vi "Recieve Idot Result utility.vi"(6 "Shots file":path=path "Z:/ShotHistory2014.txt", 7 "Log file folder":path=path "C:/Data/Shot Log.txt", 8 "error in (no error)":errorcluster, 10 "file path":path, 11 "Root Data Folder":path=path "C:/Data") -> (0 "error out":errorcluster, 2 "Formated shot data":string, 3 "File Path output":path)   [LabVIEW 2015]
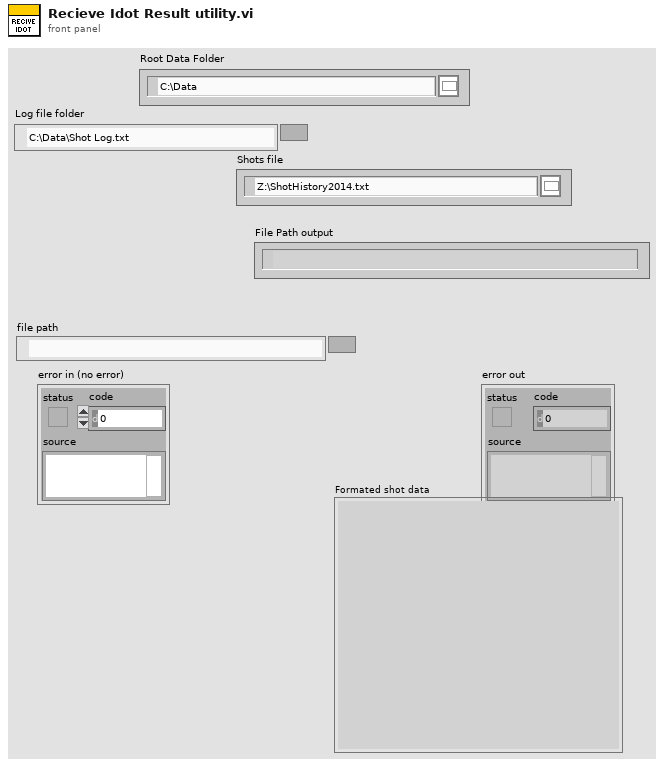
[diagram p1: front panel]
types:
  T1 = cluster{"file path":path, "Current time":timestamp, i32, dbl}
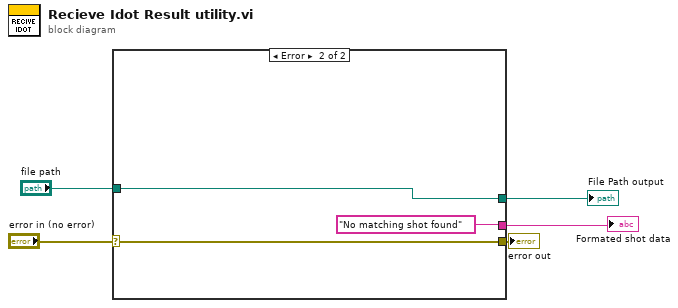
[diagram p0: block diagram]
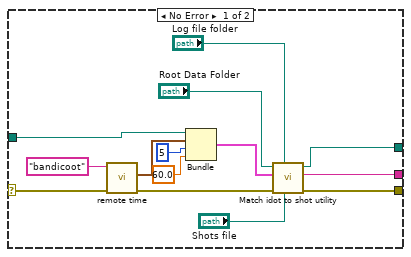
[diagram p2: hidden frame]
diagram:
  n1 = case shown="Error" "error in (no error)" {
    selector: "error in (no error)" -> [w19 w22]
    tunnel: [w10 w22] -> w4
    tunnel: [w8 w21] -> w3
    tunnel: "file path" -> [w7 w21]
    tunnel: [w6 "No matching shot found" ("Formated shot data")] -> w1
    frame No Error {
      n2 = call "remote time.vi"("Error In"=w19, "server"="bandicoot" ("command line")) -> ("Error Out"=w9:errorcluster, "Current time"=w15:timestamp)  [unwired: 6 in, 2 out]
      n3 = Bundle("file path"=w7, "Current time"=w15, 5, 60.0) -> (w14:T1)  [unwired: 1 in]
      n4 = call "Match idot to shot utility.vi"("Shots file"="Shots file", "Log file folder"="Log file folder", "error in (no error)"=w9, "Idot match record"=w14, "Root Data Folder"="Root Data Folder") -> ("error out"=w10:errorcluster, "Formated shot data"=w6:string, "File output"=w8:path)  [unwired: 4 in]
    }
    frame Error {
    }
  }
  "error out" <- w4
  "File Path output" <- w3
  "Formated shot data" <- w1
